vi "stop.vi"(8 "error in (no error)":errorcluster, 9 "CameraSettings":refnum<class "CamaraSettings.lvclass">, 10 "stop":bool, 11 "Pixelfly in":refnum<class "Pixelfly.lvclass">) -> (0 "error out":errorcluster, 1 "imageSaved":bool, 2 "stopped?":bool, 3 "Pixelfly out":refnum<class "Pixelfly.lvclass">)   [LabVIEW 2009, in "Hardware.lvlib" / "Channels.lvlib" / "Pixelfly.lvclass"]
uses:
  Pixelfly.lvclass
  Tools/CameraSettings/CamaraSettings.lvclass
  Pixelfly.lvclass/Pixelfly.ctl
  Camera.lvclass
  Tools/CameraSettings/PixelFlySettings/PixelflySettings.lvclass
  Channels.lvlib
panel:
  out "Buffer status":T1
  out "Image data":u16[][](graph)
  # "Status flags"
  # "Buffer errors"
  # "Memory usage"
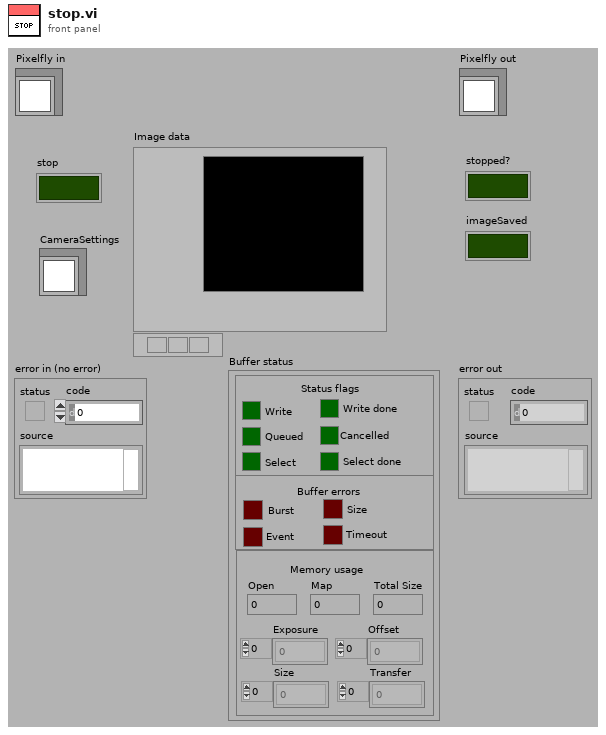
[diagram p1: front panel]
types:
  T1 = cluster{"Write":bool, "Write done":bool, "Queued":bool, "Cancelled":bool, "Select":bool, "Select done":bool, "Burst":bool, "Size":bool, "Event":bool, "Timeout":bool, "Open":i32, "Map":i32, "Exposure":i32[], "Offset":i32[], "Size":i32[], "Transfer":i32[], "Total Size":i32}
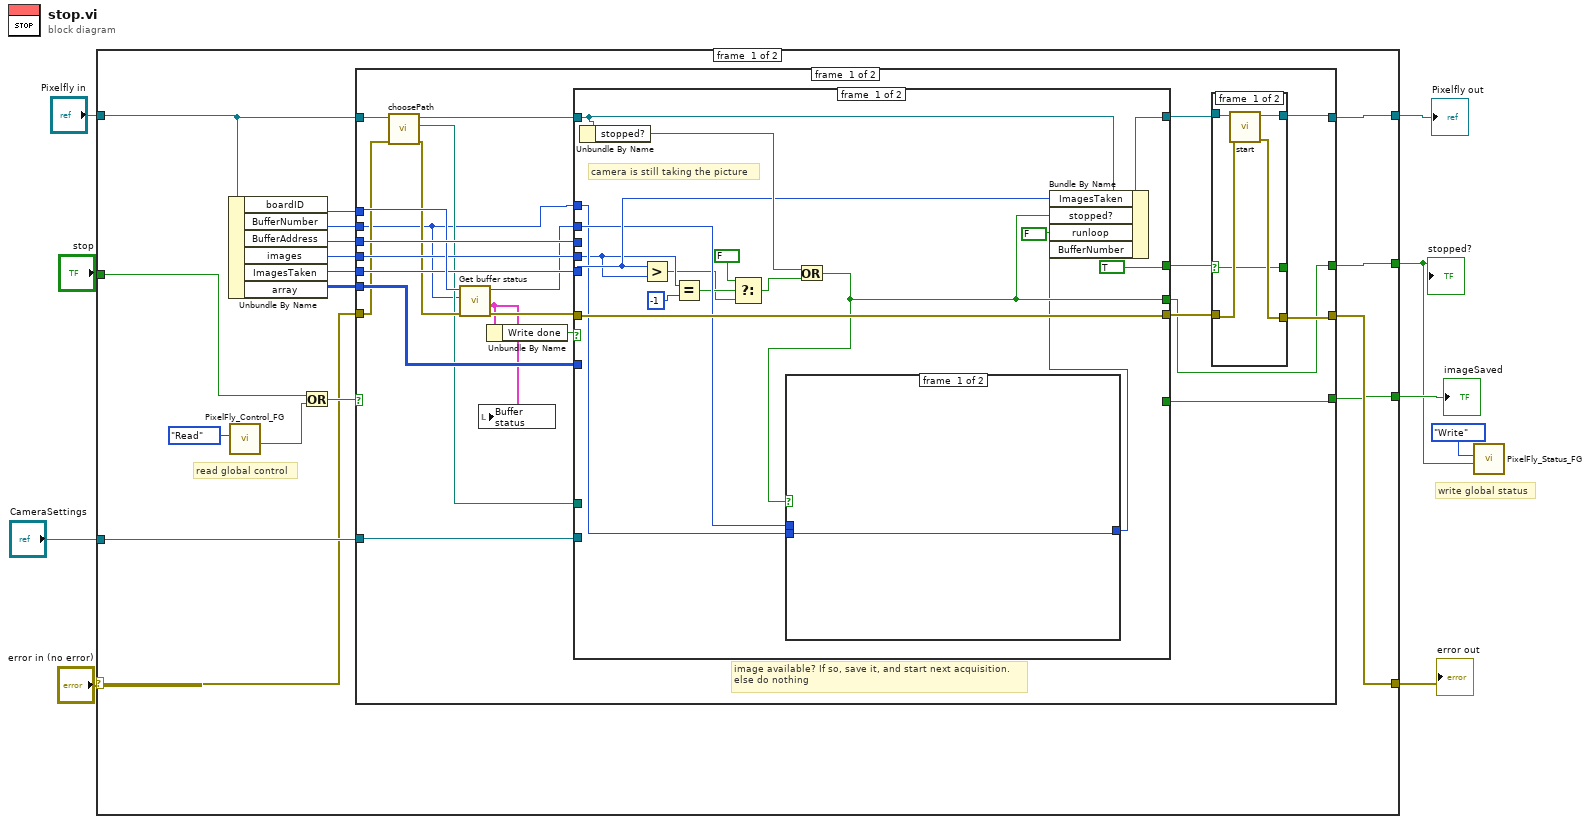
[diagram p0: block diagram]
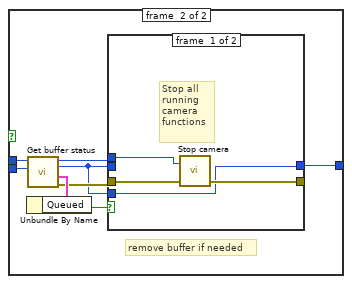
[diagram p3: hidden frame]
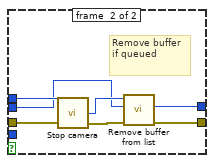
[diagram p4: hidden frame]
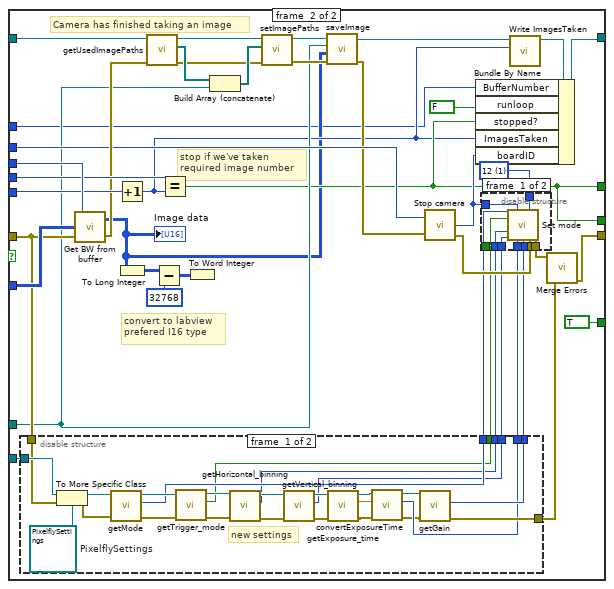
[diagram p5: hidden frame]
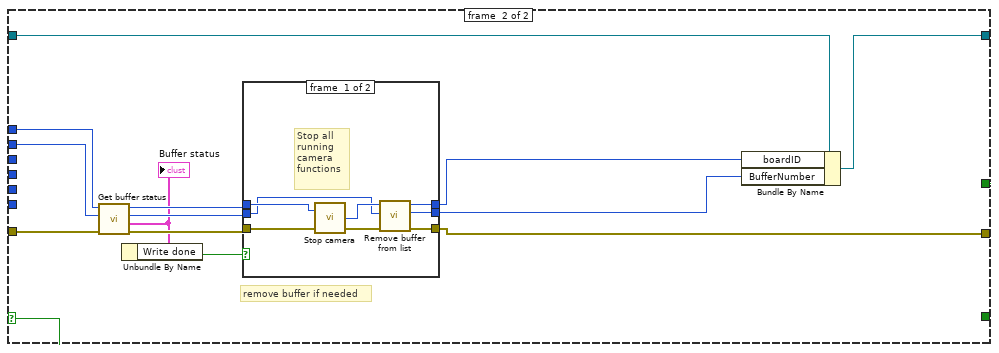
[diagram p8: hidden frame]
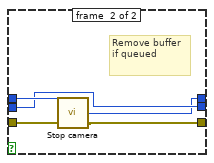
[diagram p9: hidden frame]
diagram:
  # "write global status"
  n1 = case shown="No Error" "error in (no error)" {
    selector: "error in (no error)" -> [w12 w200]
    tunnel: [w23 w200] -> w8
    tunnel: [w22 w201] -> w5
    tunnel: "Pixelfly in" -> [w26 w201]
    tunnel: "stop" -> [w13 _]
    tunnel: [w18 _] -> w1
    tunnel: "CameraSettings" -> [w16 _]
    tunnel: [w15 _] -> w3
    frame #0 {
      # "read global control"
      n2 = Unbundle By Name(w26) -> ("boardID"=w25:i32, "BufferNumber"=w24:i32, "BufferAddress"=w19:i32, "images"=w21:i32, "ImagesTaken"=w20:i32, "array"=w17:u16[][])
      n3 = call "PixelFly_Control_FG.vi"("Action"=enum16{"Write", "Read"}."Read") -> ("stopped"=w11:bool)  [unwired: 10 in]
      n4 = Or(x=w13, y=w11) -> (x .or. y?=w14:bool)
      n5 = case shown="False" w14 {
        selector: w14 -> [_ w182]
        tunnel: w26 -> [w38 w174]
        tunnel: w25 -> [w47 w186]
        tunnel: w24 -> [w28 w185]
        tunnel: w12 -> [w37 w184]
        tunnel: [w43 w183] -> w23
        tunnel: [w44 w173] -> w22
        tunnel: w21 -> [w39 _]
        tunnel: w20 -> [w41 _]
        tunnel: w19 -> [w48 _]
        tunnel: [w31 w182] -> w18
        tunnel: w17 -> [w42 _]
        tunnel: w16 -> [w33 _]
        tunnel: [w32 _] -> w15
        frame #0 {
          # "image available? If so, save it, and start next acquisition.\nelse do nothing"
          n6 = call "choosePath.vi"("error in (no error)"=w37, "Pixelfly in"=w38) -> ("error out"=w36:errorcluster, "Path"=w35:path, "Pixelfly out"=w30:refnum<class "Pixelfly.lvclass">)  [unwired: 7 in]
          n7 = call <instrlib>:"Get buffer status.vi"("error in (no error)"=w36, "Buffer request"=w28, "Handle in"=w47) -> ("error out"=w29:errorcluster, "Buffer status"=w27:T1, "Handle out"=w34:i32)  [unwired: 1 in, 1 out]
          n8 = local write "Buffer status"(w27) -> ()
          n9 = Unbundle By Name(w27) -> ("Write done"=w49:bool)
          n10 = case shown="True" w49 {
            tunnel: w48 -> [_ w135]
            tunnel: w29 -> [w74 w121]
            tunnel: [w74 w113] -> w45
            tunnel: w41 -> [w69 w134]
            tunnel: w39 -> [w63 w131]
            tunnel: [TRUE w101] -> w46
            tunnel: w42 -> [_ w133]
            tunnel: [w70 w130] -> w40
            tunnel: w35 -> [_ w105]
            tunnel: w30 -> [w71 w129]
            tunnel: w34 -> [w68 w125]
            tunnel: w33 -> [_ w122]
            tunnel: [_ TRUE] -> w32
            tunnel: [w66 w101] -> w31
            tunnel: w28 -> [w67 w95]
            frame #0 {
              # "camera is still taking the picture"
              n11 = Unbundle By Name(w71) -> ("stopped?"=w72:bool)
              n12 = Greater?(x=w69, y=w63) -> (0:w60:bool)
              n13 = Equal?(x=w63, y=-1) -> (x = y?=w62:bool)
              n14 = Select(t=FALSE, s=w62, f=w60) -> (s? t:f=w59:bool)
              n15 = Or(x=w72, y=w59) -> (x .or. y?=w66:bool)
              n16 = case shown="False" w66 {
                tunnel: w68 -> [_ w79]
                tunnel: w67 -> [w75 w78]
                tunnel: [w75 w77] -> w58
                frame #0 {
                }
                frame #1 {
                  # "remove buffer if needed"
                  n17 = call <instrlib>:"Get buffer status.vi"("Buffer request"=w78, "Handle in"=w79) -> ("error out"=w82:errorcluster, "Buffer status"=w83:T1, "Buffer number"=w76:i32, "Handle out"=w81:i32)  [unwired: 2 in]
                  n18 = Unbundle By Name(w83) -> ("Queued"=w80:bool)
                  n19 = case shown="False" w80 {
                    tunnel: w82 -> [w86 w92]
                    tunnel: [w85 w94] -> _
                    tunnel: w76 -> [_ w89]
                    tunnel: w81 -> [w87 w91]
                    tunnel: [w84 w88] -> w77
                    tunnel: w76 -> [w84 _]
                    frame #0 {
                      # "Stop all running camera functions"
                      n20 = call <instrlib>:"Stop camera.vi"("Handle in"=w87, "error in (no error)"=w86) -> ("error out"=w85:errorcluster)  [unwired: 2 out]
                    }
                    frame #1 {
                      # "Remove buffer if queued"
                      n21 = call <instrlib>:"Stop camera.vi"("Handle in"=w91, "error in (no error)"=w92) -> ("Handle out"=w90:i32, "error out"=w93:errorcluster)  [unwired: 1 out]
                      n22 = call <instrlib>:"Remove buffer from list.vi"("error in (no error)"=w93, "Buffer in"=w89, "Handle in"=w90) -> ("error out"=w94:errorcluster, "Buffer number"=w88:i32)  [unwired: 2 in, 1 out]
                    }
                  }
                }
              }
              n23 = Bundle By Name(cluster=w71, "ImagesTaken"=w69, "stopped?"=w66, "runloop"=FALSE, "BufferNumber"=w58) -> (w70:refnum<class "Pixelfly.lvclass">)
            }
            frame #1 {
              w119 = 1 items=["8", "12"] ("bits/pixel")
              # "stop if we've taken \nrequired image number"
              # "Camera has finished taking an image"
              # "convert to labview \nprefered I16 type"
              n24 = disable-structure shown="Enabled" {
                disable-tunnel: w122 -> [w152 _]
                disable-tunnel: w121 -> [w151 w161]
                disable-tunnel: [w147 _] -> w120
                disable-tunnel: [w146 _] -> w118
                disable-tunnel: [w145 _] -> w117
                disable-tunnel: [w144 _] -> w116
                disable-tunnel: [w143 _] -> w115
                disable-tunnel: [w142 w161] -> w112
                disable-tunnel: [w139 _] -> w110
                frame #0 {
                  w153 = refnum<class "PixelflySettings.lvclass"> refnum  # PixelflySettings
                  # "new settings"
                  n25 = To More Specific Class(target class=w153, reference=w152, error in=w151) -> (specific class reference=w150:refnum<class "PixelflySettings.lvclass">, error out=w149:errorcluster)
                  n26 = call "getMode.vi"("error in (no error)"=w149, "PixelflySettings in"=w150) -> ("error out"=w155:errorcluster, "mode"=w147:u16, "PixelflySettings out"=w154:refnum<class "PixelflySettings.lvclass">)  [unwired: 7 in]
                  n27 = call "getTrigger_mode.vi"("error in (no error)"=w155, "PixelflySettings in"=w154) -> ("error out"=w148:errorcluster, "trigger_mode"=w146:bool, "PixelflySettings out"=w156:refnum<class "PixelflySettings.lvclass">)  [unwired: 7 in]
                  n28 = call "getHorizontal_binning.vi"("error in (no error)"=w148, "PixelflySettings in"=w156) -> ("error out"=w158:errorcluster, "horizontal_binning"=w145:enum16{"1", "2"}, "PixelflySettings out"=w157:refnum<class "PixelflySettings.lvclass">)  [unwired: 7 in]
                  n29 = call "getVertical_binning.vi"("error in (no error)"=w158, "PixelflySettings in"=w157) -> ("error out"=w160:errorcluster, "vertical_binning"=w144:enum16{"1", "2"}, "PixelflySettings out"=w159:refnum<class "PixelflySettings.lvclass">)  [unwired: 7 in]
                  n30 = call "getExposure_time.vi"("error in (no error)"=w160, "PixelflySettings in"=w159) -> ("error out"=w138:errorcluster, "exposure_time"=w136:dbl, "PixelflySettings out"=w141:refnum<class "PixelflySettings.lvclass">)  [unwired: 7 in]
                  n31 = call "convertExposureTime.vi"("error in (no error)"=w138, "time s"=w136, "PixelflySettings in"=w141) -> ("error out"=w137:errorcluster, "exposureTime"=w139:i32, "PixelflySettings out"=w140:refnum<class "PixelflySettings.lvclass">)  [unwired: 6 in]
                  n32 = call "getGain.vi"("error in (no error)"=w137, "PixelflySettings in"=w140) -> ("error out"=w142:errorcluster, "gain"=w143:enum16{"Low", "High"})  [unwired: 7 in, 1 out]
                }
                frame #1 {
                }
              }
              n33 = call <instrlib>:"Get BW from buffer.vi"("error in (no error)"=w121, "Array input"=w133, "Buffer address"=w135) -> ("error out"=w128:errorcluster, "Image data"=w97:u16[][])
              "Image data" <- w97
              n34 = Increment(x=w134) -> (x+1=w98:i32)
              n35 = To Long Integer(number=w97) -> (32bit integer=w103:i32[][])
              n36 = call "getUsedImagePaths.vi"("error in (no error)"=w128, "Camera in"=w129) -> ("error out"=w109:errorcluster, "UsedImagePaths"=w126:path[], "Camera out"=w127:refnum<class "Pixelfly.lvclass">)  [unwired: 7 in]
              n37 = Subtract(x=w103, y=32768) -> (x-y=w104:i32[][])
              n38 = Equal?(x=w131, y=w98) -> (x = y?=w101:bool)
              n39 = To Word Integer(number=w104) -> ()  [unwired: 1 out]
              n40 = Build Array (concatenate)(w126, w105) -> (w132:path[])
              n41 = call "setImagePaths.vi"("error in (no error)"=w109, "ImagePaths"=w132, "Camera in"=w127) -> ("error out"=w107:errorcluster, "Camera out"=w108:refnum<class "Pixelfly.lvclass">)  [unwired: 7 in]
              n42 = call "saveImage.vi"("error in (no error)"=w107, "I16bit image data"=w97, "Path"=w105, "Pixelfly in"=w108) -> ("error out"=w106:errorcluster, "Pixelfly out"=w100:refnum<class "Pixelfly.lvclass">)  [unwired: 6 in]
              n43 = call <instrlib>:"Stop camera.vi"("Handle in"=w125, "error in (no error)"=w106) -> ("Handle out"=w124:i32, "error out"=w123:errorcluster)  [unwired: 1 out]
              n44 = disable-structure shown="Enabled" {
                disable-tunnel: w124 -> [w171 _]
                disable-tunnel: w123 -> [w170 w172]
                disable-tunnel: w120 -> [w169 _]
                disable-tunnel: w119 -> [w168 _]
                disable-tunnel: w118 -> [w167 _]
                disable-tunnel: w117 -> [w166 _]
                disable-tunnel: w116 -> [w165 _]
                disable-tunnel: w115 -> [w164 _]
                disable-tunnel: [w163 w172] -> w114
                disable-tunnel: w110 -> [w162 _]
                frame #0 {
                  n45 = call <instrlib>:"Set mode.vi"("Exposure mode"=w169, "Handle in"=w171, "bits/pixel"=w168, "trigger"=w167, "H bin"=w166, "V bin"=w165, "exp time"=w162, "gain"=w164, "error in (no error)"=w170) -> ("error out"=w163:errorcluster)  [unwired: 6 in]
                }
                frame #1 {
                }
              }
              n46 = call "Write ImagesTaken.vi"("ImagesTaken"=w98, "Camera in"=w100) -> ("Camera out"=w99:refnum<class "Pixelfly.lvclass">)  [unwired: 8 in, 1 out]
              n47 = Bundle By Name(cluster=w99, "BufferNumber"=w95, "runloop"=FALSE, "stopped?"=w101, "ImagesTaken"=w98, "boardID"=w124) -> (w130:refnum<class "Pixelfly.lvclass">)
              n48 = call <vilib>:"Merge Errors.vi"("error in 2 (no error)"=w112, "error in 1 (no error)"=w114) -> ("error out"=w113:errorcluster)  [unwired: 5 in]
            }
          }
          n49 = case shown="False" w46 {
            selector: w46 -> [w51 w56]
            tunnel: w45 -> [w53 w57]
            tunnel: [w54 w55] -> w44
            tunnel: [w52 w57] -> w43
            tunnel: [w51 w56] -> _
            tunnel: w40 -> [w50 w55]
            frame #0 {
              n50 = call-dynamic "start.vi"("error in (no error)"=w53, "Pixelfly in"=w50) -> ("error out"=w52:errorcluster, "Pixelfly out"=w54:refnum<class "Pixelfly.lvclass">)  [unwired: 8 in]
            }
            frame #1 {
            }
          }
        }
        frame #1 {
          # "remove buffer if needed"
          n51 = call <instrlib>:"Get buffer status.vi"("error in (no error)"=w184, "Buffer request"=w185, "Handle in"=w186) -> ("error out"=w181:errorcluster, "Buffer status"=w177:T1, "Buffer number"=w180:i32, "Handle out"=w179:i32)  [unwired: 1 in]
          "Buffer status" <- w177
          n52 = Unbundle By Name(w177) -> ("Write done"=w178:bool)
          n53 = case shown="True" w178 {
            tunnel: w181 -> [w193 w199]
            tunnel: [w191 w197] -> w183
            tunnel: w180 -> [w189 w196]
            tunnel: w179 -> [w194 w198]
            tunnel: [w188 w196] -> w175
            tunnel: [w187 w195] -> w176
            frame #0 {
              # "Stop all running camera functions"
              n54 = call <instrlib>:"Stop camera.vi"("Handle in"=w194, "error in (no error)"=w193) -> ("Handle out"=w190:i32, "error out"=w192:errorcluster)  [unwired: 1 out]
              n55 = call <instrlib>:"Remove buffer from list.vi"("error in (no error)"=w192, "Buffer in"=w189, "Handle in"=w190) -> ("error out"=w191:errorcluster, "Buffer number"=w188:i32, "Handle out"=w187:i32)  [unwired: 2 in]
            }
            frame #1 {
              # "Remove buffer if queued"
              n56 = call <instrlib>:"Stop camera.vi"("Handle in"=w198, "error in (no error)"=w199) -> ("Handle out"=w195:i32, "error out"=w197:errorcluster)  [unwired: 1 out]
            }
          }
          n57 = Bundle By Name(cluster=w174, "boardID"=w176, "BufferNumber"=w175) -> (w173:refnum<class "Pixelfly.lvclass">)
        }
      }
    }
    frame #1 {
    }
  }
  "error out" <- w8
  "Pixelfly out" <- w5
  "stopped?" <- w1
  "imageSaved" <- w3
  n58 = call "PixelFly_Status_FG.vi"("stop"=w1, "Action"=enum16{"Write", "Read"}."Write") -> ()  [unwired: 9 in, 1 out]
